vi "zmq device.vi"(8 "error in (no error)":errorcluster, 9 "backend_":u32, 10 "frontend_":u32, 11 "type_":i32) -> (0 "error out":errorcluster, 1 "backend_ out":u32, 2 "frontend_ out":u32, 3 "function return":i32)   [LabVIEW 2025, in "libzmq-v143-mt-4_3_6.lvlib"]
doc: "ZMQ_EXPORT int zmq_device (int type_, void *frontend_, void *backend_);"
uses:
  libzmq-v143-mt-4_3_6.lvlib
  LV/LibZMQ/libzmq/lv_x86/bin/Release/libzmq-v143-mt-4_3_6.dll
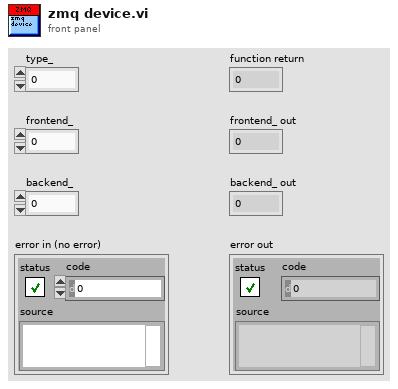
[diagram p1: front panel]
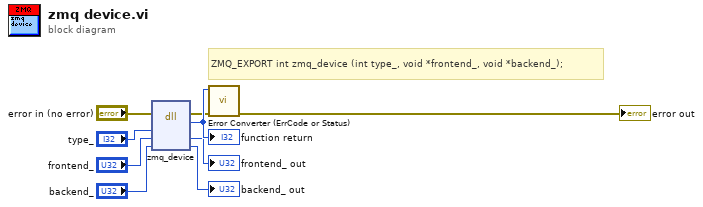
[diagram p0: block diagram]
diagram:
  # "ZMQ_EXPORT int zmq_device (int type_, void *frontend_, void *backend_);"
  n1 = dll-call lib="C:/LV/LibZMQ/libzmq/lv_x86/bin/Release/libzmq-v143-mt-4_3_6.*" fn="zmq_device"(error in="error in (no error)", "type_"="type_", "frontend_"="frontend_", "backend_"="backend_") -> (error out=w2:errorcluster, w9:i32, "frontend_"=→"frontend_ out":u32, "backend_"=→"backend_ out":u32)  [unwired: 3 in, 1 out]
  "function return" <- w9
  n2 = call "Error Converter (ErrCode or Status).vi"("error in (no error)"=w2, "error code"=w9) -> ("error out"=→"error out":errorcluster)  [unwired: 9 in]
